vi "format_chart.vi"() -> ()   [LabVIEW 2020]
panel:
  in  "Chart Ref In":refnum<vi>
  out "Chart Ref Out":refnum<vi>
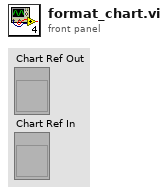
[diagram p1: front panel]
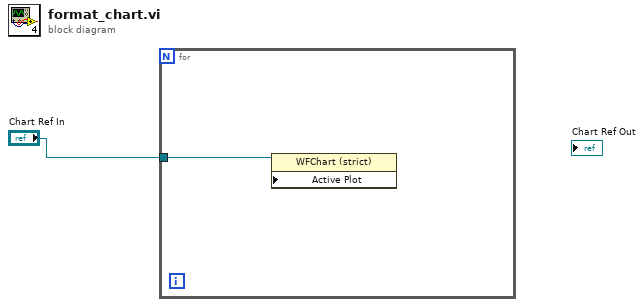
[diagram p0: block diagram]
diagram:
  n1 = for {
    tunnel: "Chart Ref In" -> [w2]
    n2 = property class="WFChart (strict)" props=["Active Plot"](reference=w2) -> ()  [unwired: 2 in, 2 out]
  }
